vi "Can I Reach Destination.vi"(4 "Max Elevation per step":i32, 5 "Elevation Grid Numeric":i32[][](array[numeric]), 6 "Destination Location":cdb, 9 "Current Location":cdb) -> (3 "Can I reach Destination ?":bool)   [LabVIEW 2020, in "AoC 2022.lvlib"]
uses:
  AoC 2022.lvlib
  a076882e-ba63-4d2e-bd81-09dae0a55d11.vi
  8b9bf59d-da71-4f8a-b94f-04aaeca68a64.vi
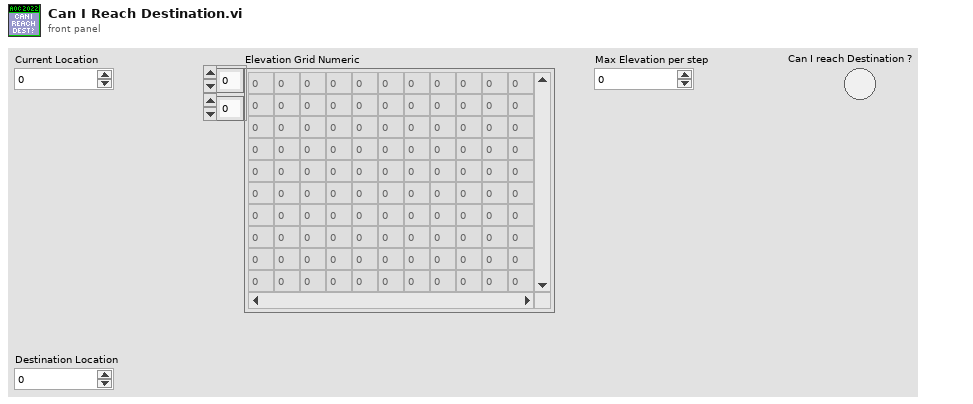
[diagram p1: front panel]
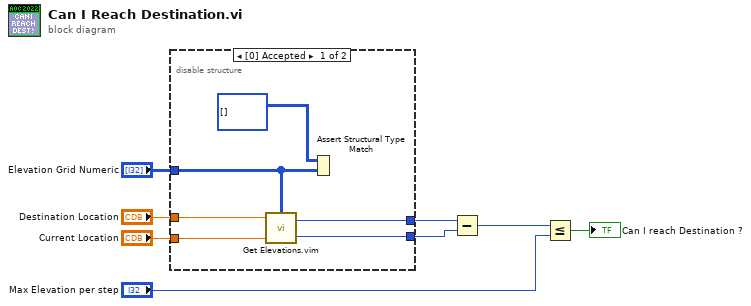
[diagram p0: block diagram]
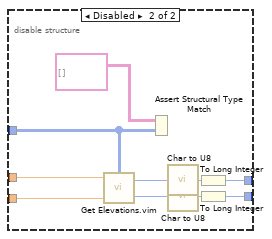
[diagram p2: hidden frame]
diagram:
  n1 = disable-structure shown="[0] Accepted" {
    disable-tunnel: "Destination Location" -> [w14 w22]
    disable-tunnel: "Current Location" -> [w13 w21]
    disable-tunnel: "Elevation Grid Numeric" -> [w10 w18]
    disable-tunnel: [w12 w16] -> w8
    disable-tunnel: [w11 w15] -> w3
    frame Enabled {
      n2 = call "Get Elevations.vim"("Elevation Grid Numeric"=w10, "Current Location"=w13, "Destination Location"=w14) -> ("Current Elevation"=w11:i32, "Destination Elevation"=w12:i32)  [unwired: 1 in]
      n3 = Assert Structural Type Match(0:w10, 1:i32[][] []) -> ()
    }
    frame Disabled {
      n4 = call "Get Elevations.vim"("Elevation Grid Numeric"=w18, "Current Location"=w21, "Destination Location"=w22) -> ("Current Elevation"=w19:i32, "Destination Elevation"=w20:i32)  [unwired: 1 in]
      n5 = Assert Structural Type Match(0:w18, 1:string[][] []) -> ()
      n6 = call "Char to U8.vi"("Char"=w20) -> ("U8"=w24:u8)
      n7 = call "Char to U8.vi"("Char"=w19) -> ("U8"=w23:u8)
      n8 = To Long Integer(number=w24) -> (32bit integer=w16:i32)
      n9 = To Long Integer(number=w23) -> (32bit integer=w15:i32)
    }
  }
  n10 = Subtract(x=w8, y=w3) -> (x-y=w6:i32)
  n11 = Less Or Equal?(x=w6, y="Max Elevation per step") -> (x <= y?=→"Can I reach Destination ?":bool)
